vi "MovingAvg.vi"(0 "입력":dbl, 1 "이동평균을 구할 자료의 개수":u16) -> (2 "이동평균을 구하는데 사용된 배열":dbl[](array[numeric]), 3 "합계":dbl, 4 "이동평균":dbl)   [LabVIEW 2020]
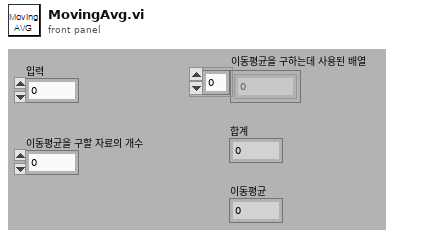
[diagram p1: front panel]
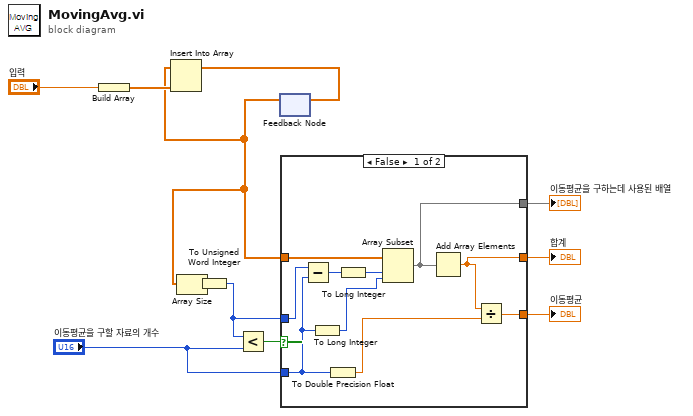
[diagram p0: block diagram]
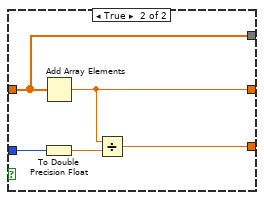
[diagram p2: hidden frame]
diagram:
  n1 = Build Array("입력") -> (w3:dbl[])
  n2 = feedback #1() -> (w1:dbl[])  [unwired: 1 in]
  n3 = Insert Into Array(array=w1, new element=w3) -> (w2:dbl[])  [unwired: 1 in]
  n4 = Array Size(array=w1) -> (size(s)=w6:i32)
  n5 = To Unsigned Word Integer(number=w6) -> (unsigned 16bit integer=w4:u16)
  n6 = Less?(x=w4, y="이동평균을 구할 자료의 개수") -> (x < y?=w11:bool)
  n7 = feedback-in #1(w2) -> ()
  n8 = case shown="False" w11 {
    tunnel: w1 -> [w14 w22]
    tunnel: [w21 w24] -> w10
    tunnel: w4 -> [w16 w26]
    tunnel: [w19 w23] -> w9
    tunnel: [w18 w22] -> w8
    tunnel: "이동평균을 구할 자료의 개수" -> [w15 _]
    frame False {
      n9 = Subtract(x=w16, y=w15) -> (x-y=w17:u16)
      n10 = To Long Integer(number=w15) -> (32bit integer=w12:i32)
      n11 = To Double Precision Float(number=w15) -> (double precision float=w20:dbl)
      n12 = To Long Integer(number=w17) -> (32bit integer=w13:i32)
      n13 = Array Subset(array=w14, index=w13, length=w12) -> (w18:dbl[])
      n14 = Add Array Elements(numeric array=w18) -> (sum=w21:dbl)
      n15 = Divide(x=w21, y=w20) -> (x/y=w19:dbl)
    }
    frame True {
      n16 = Add Array Elements(numeric array=w22) -> (sum=w24:dbl)
      n17 = To Double Precision Float(number=w26) -> (double precision float=w25:dbl)
      n18 = Divide(x=w24, y=w25) -> (x/y=w23:dbl)
    }
  }
  "이동평균을 구하는데 사용된 배열" <- w8
  "합계" <- w10
  "이동평균" <- w9
